vi "Execute Multiple Commands with Multiple Channels.vi"() -> ()   [LabVIEW 2018]
doc: "Executes multiple, sequential commands using a separate channel for each command on a remote SSH server. This is similar to executing multiple commands over SSH with each command as a separate command line instruction."
uses:
  Toolkit/Session/Support/Password Authentication.vi
  Toolkit/Channel/Support/Create from Session.vi
  Toolkit/Channel/Support/Destroy to Session.vi
  Toolkit/SSH/SSH.lvclass
  Toolkit/Session/Session.lvclass
  Toolkit/Channel/Channel.lvclass
panel:
  out "Response 2":string
  in  "Command 2":string="echo \"Hello World from the second command!\""
  out "Response 1":string
  in  "Command 1":string="echo \"Hello World from the first command!\""
  in  "Remote SSH Server":string
  in  "Password":string
  in  "Username":string
  # "Overview: Demonstrates executing multiple, sequential commands on a remote SSH server using multiple, different channels for each command\nInstructions:\n1. Enter the IP address or host name of the remote SSH server. This can be a CompactRIO (cRIO) running the National Instruments Linux Real-Time (NI Linux RT) operating system with the Enable Secure Shell Server (sshd) checkbox checked. \n2. Enter a username. If using a cRIO with a default configuration, then the username is \"admin\".\n3. Enter a password for the username. If using a cRIO with a default configuration, then the password is blank (empty).\n4. Run this VI.\n5. Observe \"Hello World from the first command!\" and \"Hellow World from the second command!\" in Response 1 and Response 2 indicators, respectivelu.\n6. Change the two commands,\n7. Run this VI again.\n8. Observe the responses for the two commands"
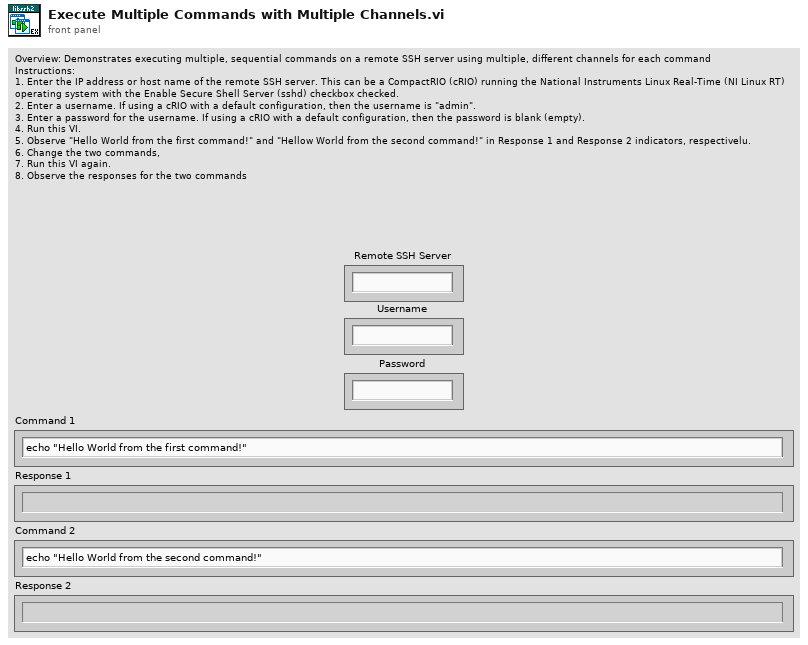
[diagram p1: front panel]
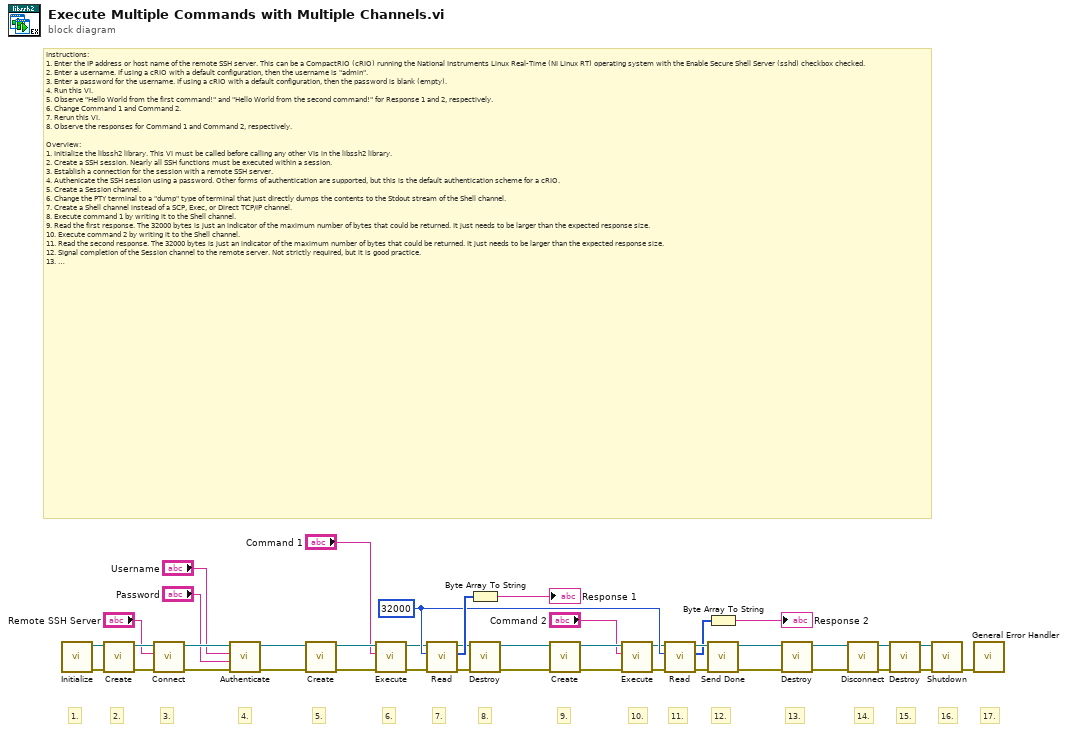
[diagram p0: block diagram]
diagram:
  w16 = u64 32000 ("Max Data Length")
  # "17."
  # "16."
  # "15."
  # "14."
  # "13."
  # "12."
  # "11."
  # "10."
  # "9."
  # "8."
  # "7."
  # "6."
  # "5."
  # "4."
  # "3."
  # "2."
  # "1."
  # "Instructions:\n1. Enter the IP address or host name of the remote SSH server. This can be a CompactRIO (cRIO) running the National Instruments Linux Real-Time (NI Linux RT) operating system with the Enable Secure Shell Server (sshd) checkbox checked. \n2. Enter a username. If using a cRIO with a default configuration, then the username is \"admin\".\n3. Enter a password for the username. If using a cRIO with a default configuration, then the password is blank (empty).\n4. Run this VI.\n5. Observe \"Hello World from the first command!\" and \"Hello World from the second command!\" for Response 1 and 2, respectively.\n6. Change Command 1 and Command 2.\n7. Rerun this VI.\n8. Observe the responses for Command 1 and Command 2, respectively.\n\nOverview:\n1. Initialize the libssh2 library. This VI must be called before calling any other VIs in the libssh2 library.\n2. Create a SSH session. Nearly all SSH functions must be executed within a session.\n3. Establish a connection for the session with a remote SSH server.\n4. Authenicate the SSH session using a password. Other forms of authentication are supported, but this is the default authentication scheme for a cRIO. \n5. Create a Session channel.\n6. Change the PTY terminal to a \"dump\" type of terminal that just directly dumps the contents to the Stdout stream of the Shell channel.\n7. Create a Shell channel instead of a SCP, Exec, or Direct TCP/IP channel.\n8. Execute command 1 by writing it to the Shell channel.\n9. Read the first response. The 32000 bytes is just an indicator of the maximum number of bytes that could be returned. It just needs to be larger than the expected response size.\n10. Execute command 2 by writing it to the Shell channel.\n11. Read the second response. The 32000 bytes is just an indicator of the maximum number of bytes that could be returned. It just needs to be larger than the expected response size.\n12. Signal completion of the Session channel to the remote server. Not strictly required, but it is good practice. \n13. Destroy the Session channel. Since the \"Create\" VI is used, the complementary \"Destroy\" VI must be used to free resources within the libssh2 library. \n14. Disconnect from the remote SSH server.\n15. Destroy the session to free resources within the libssh2 library.\n16. Shutdown the libssh2 library. This VI must be last VI called for the libssh2 library. No other libssh2 VIs should be called once this VI is executed.\n17. Provide some error handling and reporting. Libssh2 errors will be in the -8100 range."
  n1 = call "Initialize.vi"() -> ("Error Out"=w40:errorcluster, "SSH"=w41:refnum<class "SSH.lvclass">)  [unwired: 10 in]
  n2 = call "Create.vi"("Error In"=w40, "SSH"=w41) -> ("Error Out"=w38:errorcluster, "Sesssion"=w39:refnum<class "Session.lvclass">)  [unwired: 8 in]
  n3 = call "Connect.vi"("Error In"=w38, "Address"="Remote SSH Server", "Session In"=w39) -> ("Error Out"=w36:errorcluster, "Sesssion Out"=w37:refnum<class "Session.lvclass">)  [unwired: 7 in]
  n4 = call-poly "Authenticate.vi"("Error In"=w36, "Password"="Password", "Username"="Username", "Session In"=w37) -> ("Error Out"=w34:errorcluster, "Sesssion Out"=w35:refnum<class "Session.lvclass">)  [unwired: 6 in]
  n5 = call-poly "Create.vi"("Error In"=w34, "Session"=w35) -> ("Error Out"=w13:errorcluster, "Channel"=w14:refnum<class "Channel.lvclass">)  [unwired: 8 in]
  n6 = call "Execute.vi"("Error In"=w13, "Command"="Command 1", "Channel In"=w14) -> ("Error Out"=w10:errorcluster, "Channel Out"=w11:refnum<class "Channel.lvclass">)  [unwired: 7 in]
  n7 = call "Read.vi"("Error In"=w10, "Max Data Length"=w16, "Channel In"=w11) -> ("Error Out"=w8:errorcluster, "Data"=w25:u8[], "Channel Out"=w9:refnum<class "Channel.lvclass">)  [unwired: 6 in]
  n8 = Byte Array To String(unsigned byte array=w25) -> (string=→"Response 1":string)
  n9 = call-poly "Destroy.vi"("Error In"=w8, "Channel"=w9) -> ("Error Out"=w7:errorcluster, "Session"=w6:refnum<class "Session.lvclass">)  [unwired: 8 in]
  n10 = call-poly "Create.vi"("Error In"=w7, "Session"=w6) -> ("Error Out"=w2:errorcluster, "Channel"=w5:refnum<class "Channel.lvclass">)  [unwired: 8 in]
  n11 = call "Execute.vi"("Error In"=w2, "Command"="Command 2", "Channel In"=w5) -> ("Error Out"=w3:errorcluster, "Channel Out"=w4:refnum<class "Channel.lvclass">)  [unwired: 7 in]
  n12 = call "Read.vi"("Error In"=w3, "Max Data Length"=w16, "Channel In"=w4) -> ("Error Out"=w18:errorcluster, "Data"=w15:u8[], "Channel Out"=w17:refnum<class "Channel.lvclass">)  [unwired: 6 in]
  n13 = Byte Array To String(unsigned byte array=w15) -> (string=→"Response 2":string)
  n14 = call "Send Done.vi"("Error In"=w18, "Channel In"=w17) -> ("Error Out"=w32:errorcluster, "Channel Out"=w33:refnum<class "Channel.lvclass">)  [unwired: 8 in]
  n15 = call-poly "Destroy.vi"("Error In"=w32, "Channel"=w33) -> ("Error Out"=w30:errorcluster, "Session"=w31:refnum<class "Session.lvclass">)  [unwired: 8 in]
  n16 = call "Disconnect.vi"("Error In"=w30, "Session In"=w31) -> ("Error Out"=w28:errorcluster, "Sesssion Out"=w29:refnum<class "Session.lvclass">)  [unwired: 8 in]
  n17 = call "Destroy.vi"("Error In"=w28, "Session"=w29) -> ("Error Out"=w26:errorcluster, "SSH"=w27:refnum<class "SSH.lvclass">)  [unwired: 8 in]
  n18 = call "Shutdown.vi"("Error In"=w26, "SSH"=w27) -> ("Error Out"=w20:errorcluster)  [unwired: 9 in]
  n19 = call <vilib>:"General Error Handler.vi"("error in (no error)"=w20) -> ()  [unwired: 10 in, 5 out]
